vi "ReadArea.vi"() -> ()   [LabVIEW 2014]
uses:
  lib/Snap7.lvlib
panel:
  out "?":string
  out "ASCII Data":string
  out "Hex Data":string
  out "Running":bool
  out "Status":string="No Error"
  in  "Word Length":i32(ring)=2 items=["Bit"=1, "Byte"=2, "Word"=4, "DWord"=6, "Real"=8, "Counter"=28, "Timer"=29]
  in  "Area":i32(ring)=132 items=["Inputs (EB)"=129, "Output (AB)"=130, "Bit Memory (M)"=131, "Data (DB)"=132, "Counters (Z)"=28, "Timers (T)"=29]
  in  "Amount":i32=50
  in  "Start":i32
  in  "DB Number":i32=5
  out "Data":u8[](array[numeric])
  in  "?":bool
  in  "Slot":i32
  in  "Rack":i32
  in  "Address IP":string="192.168.0.30"
  # "Data Read"
  # "ISO : An error occurred during send TCP : Connection reset by peer"
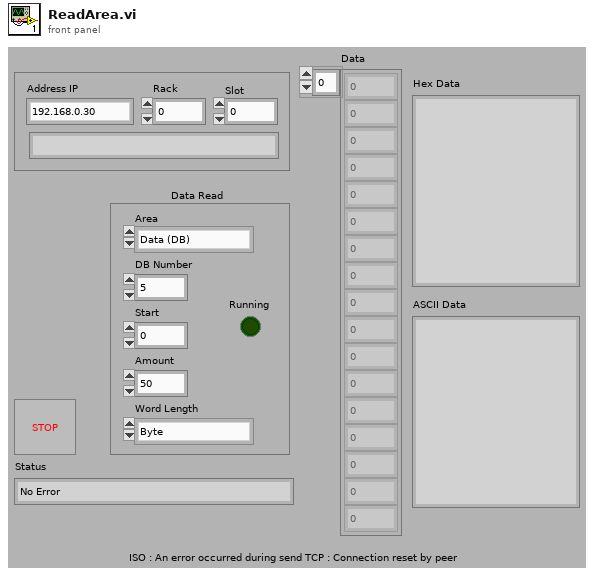
[diagram p1: front panel]
types:
  T1 = enum16{"big-endian, network order", "native, host order", "little-endian"}
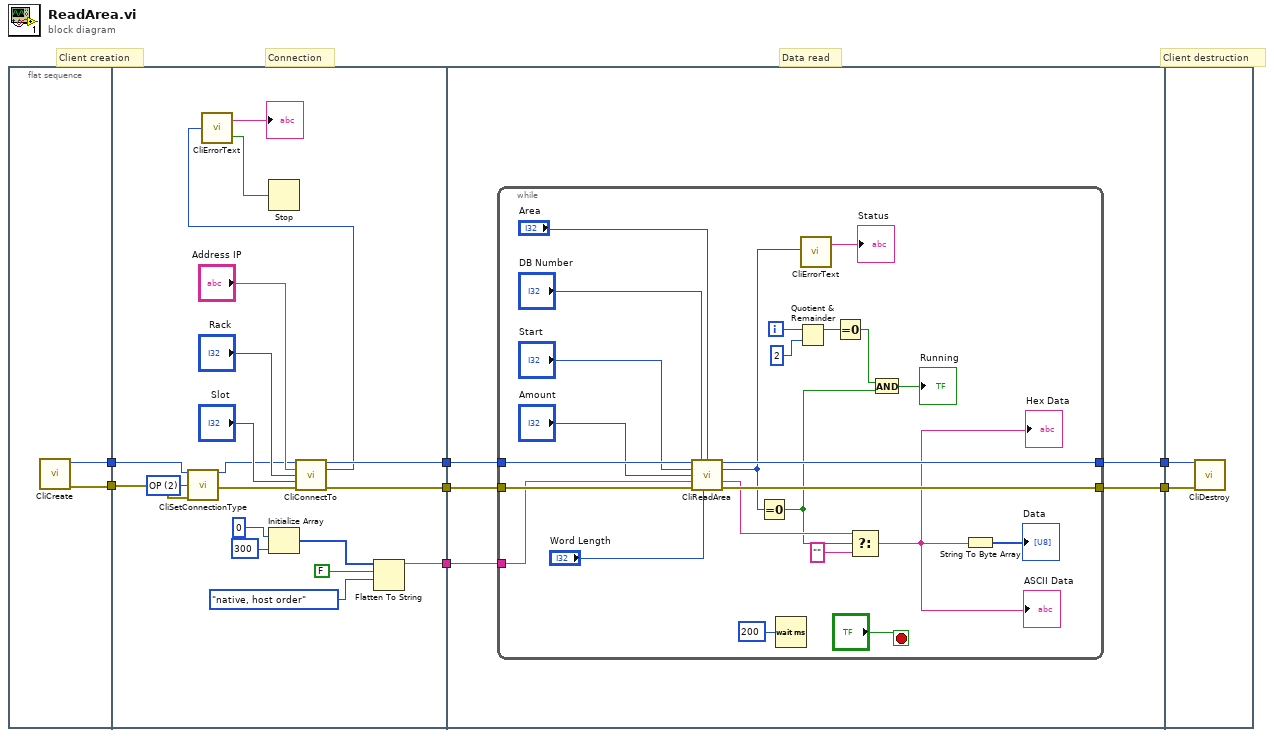
[diagram p0: block diagram]
diagram:
  # "Client destruction"
  # "Data read"
  # "Connection"
  # "Client creation"
  n1 = flat-sequence {
    tunnel: [w9] -> w4
    tunnel: [w8] -> w3
    tunnel: [w23] -> w7
    tunnel: [w18] -> w6
    tunnel: [w22] -> w5
    tunnel: w4 -> [w12]
    tunnel: w3 -> [w14]
    tunnel: w7 -> [w33]
    tunnel: w6 -> [w32]
    tunnel: w5 -> [w31]
    tunnel: [w30] -> w2
    tunnel: [w29] -> w1
    tunnel: w2 -> [w59]
    tunnel: w1 -> [w58]
    frame #0 {
      n2 = call "CliCreate.vi"() -> ("ref out"=w9:u64, "error out"=w8:errorcluster)  [unwired: 14 in]
    }
    frame #1 {
      w10 = u16 2 items=["PG"=1, "OP"=2, "S7 Basic"=3] ("ConnectionType")
      n3 = call "CliSetConnectionType.vi"("ref in"=w12, "ConnectionType"=w10, "error in (no error)"=w14) -> ("ref out"=w11:u64, "error out"=w13:errorcluster)  [unwired: 10 in, 1 out]
      n4 = Initialize Array(u8 0, 300) -> (w26:u8[])
      n5 = call "CliConnectTo.vi"("ref in"=w11, "Address"="Address IP", "Rack"="Rack", "Slot"="Slot", "error in (no error)"=w13) -> ("ref out"=w18:u64, "Result"=w15:i32, "error out"=w23:errorcluster)  [unwired: 8 in]
      n6 = call "CliErrorText.vi"("ErrNo"=w15) -> ("Error"=w16:bool, "ErrMessage"=→"?":string)
      n7 = Stop(stop? (T)=w16) -> ()
      n8 = Flatten To String(anything=w26, prepend array or string size? (T)=FALSE, byte order (0:big-endian, network order)=T1."native, host order") -> (data string=w22:string)  [unwired: 1 in, 2 out]
    }
    frame #2 {
      n9 = while {
        tunnel: w33 -> [w55]
        tunnel: w32 -> [w54]
        tunnel: w31 -> [w53]
        tunnel: [w47] -> w30
        tunnel: [w46] -> w29
        i -> [w44]
        stop <- "?" stop-if-true
        n10 = call "CliReadArea.vi"("ref in"=w54, "DB Number"="DB Number", "Area"="Area", "Start"="Start", "Amount"="Amount", "data in"=w53, "error in (no error)"=w55, "Word Length"="Word Length") -> ("ref out"=w47:u64, "Result"=w45:i32, "data out"=w38:string, "error out"=w46:errorcluster)  [unwired: 4 in]
        n11 = Equal To 0?(x=w45) -> (x = 0?=w37:bool)
        n12 = Wait (ms)(milliseconds to wait=u32 200 ("Loop Delay (ms)")) -> ()  [unwired: 1 out]
        n13 = Quotient & Remainder(x=w44, y=2) -> (x-y*floor(x/y)=w42:i32)  [unwired: 1 out]
        n14 = call "CliErrorText.vi"("ErrNo"=w45) -> ("ErrMessage"=→"Status":string)  [unwired: 1 out]
        n15 = Equal To 0?(x=w42) -> (x = 0?=w41:bool)
        n16 = Select(t=w38, s=w37, f="") -> (s? t:f=w35:string)
        "ASCII Data" <- w35
        "Hex Data" <- w35
        n17 = And(x=w41, y=w37) -> (x .and. y?=→"Running":bool)
        n18 = String To Byte Array(string=w35) -> (unsigned byte array=→"Data":u8[])
      }
    }
    frame #3 {
      n19 = call "CliDestroy.vi"("ref in"=w59, "error in (no error)"=w58) -> ()  [unwired: 13 in, 1 out]
    }
  }
